vi "Write Timeout (ms).vi"(8 "error in (no error)":errorcluster, 10 "Timeout (ms)":i32=100, 11 "FPGA Serial Session in":refnum<class "FPGA Serial Session.lvclass">) -> (0 "error out":errorcluster, 3 "FPGA Serial Session out":refnum<class "FPGA Serial Session.lvclass">)   [LabVIEW 2015, in "FPGA Serial Session.lvclass"]
uses:
  FPGA Serial Session.lvclass
  FPGA Serial Session.lvclass/FPGA Serial Session.ctl
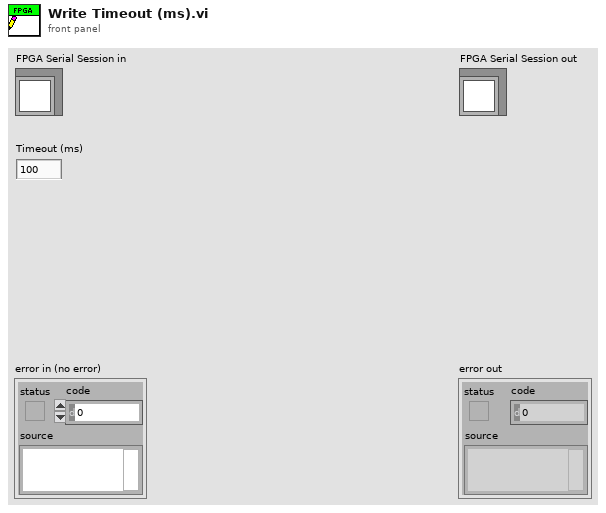
[diagram p1: front panel]
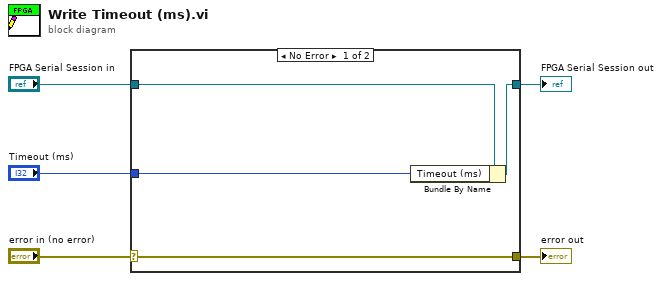
[diagram p0: block diagram]
diagram:
  n1 = case shown="No Error" "error in (no error)" {
    selector: "error in (no error)" -> [w9 w10]
    tunnel: [w9 w10] -> w4
    tunnel: [w7 w11] -> w2
    tunnel: "FPGA Serial Session in" -> [w8 w11]
    tunnel: "Timeout (ms)" -> [w6 _]
    frame No Error {
      n2 = Bundle By Name(cluster=w8, "Timeout (ms)"=w6) -> (w7:refnum<class "FPGA Serial Session.lvclass">)
    }
    frame Error {
    }
  }
  "error out" <- w4
  "FPGA Serial Session out" <- w2
